vi "HostCurrentTimeGLOBAL (1).vi"() -> ()   [LabVIEW 2017]
panel:
  in  "CurrentTime":dbl
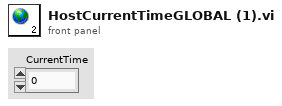
[diagram p1: front panel]
diagram:
